vi "Think 3.vi"(2 "World (mapped) in":i8[][](array[numeric]), 3 "E":i8, 4 "Sense Heading":i8, 5 "Sensor View":i8[][](array[numeric]), 6 "Y":i8, 7 "X":i8) -> (0 "World (mapped) out":i8[][](array[numeric]), 1 "V Heading":i8)   [LabVIEW 2014]
doc: "This VI takes in the current location of the robot (X,Y), the 3x3 sensor reading of the surrounding area, and the direction of the highest-valued neighboring food source."
uses:
  <vilib>/imath/engines/lvmath2/RunTimeEngine/BuiltInFunctions/findnz/NIMS_[3o]_findnz(GM).vi
  <instcachedir>/0/NIMS_[3o]_findnz(GM)_AD3DA0EED2E643EC9DE9AF9EC032A43D.lvgen/NIMS_[3o]_findnz(GM)_AD3DA0EED2E643EC9DE9AF9EC032A43D_003.vi
  <vilib>/imath/engines/lvmath2/RunTimeEngine/BuiltInFunctions/length/NIMS_length(GM).vi
  <instcachedir>/0/NIMS_length(GM)_47CEC356FCE0482D9BA47DC61C99F2C7.lvgen/NIMS_length(GM)_47CEC356FCE0482D9BA47DC61C99F2C7_001.vi
  <vilib>/imath/engines/lvmath2/RunTimeEngine/RangeToken/NIMS_Range_R2 - Integer.vi
  <instcachedir>/0/NIMS_Range_R2 - Integer_2D1304BAF97744E0A293025746CBADFC.lvgen/NIMS_Range_R2 - Integer_2D1304BAF97744E0A293025746CBADFC_000.vi
  <vilib>/imath/engines/lvmath2/RunTimeEngine/CommandStatement/MC_CommandStatement_break.vi
  <vilib>/imath/engines/lvmath2/RunTimeEngine/VariableToken/NIMS_VariableToken_CondDefinedDefinedByReplace.vi
  <instcachedir>/0/NIMS_VariableToken_CondDefinedDefinedByReplace_D162CFFC24174562A9FEA619A91E1A56.lvgen/NIMS_VariableToken_CondDefinedDefinedByReplace_D162CFFC24174562A9FEA619A91E1A56_002.vi
  <vilib>/imath/engines/lvmath2/RunTimeEngine/IndexRead/NIMS M(S).vi
  <instcachedir>/0/NIMS M(S)_B826C018497E4940AE96BD27B540B6FB.lvgen/NIMS M(S)_B826C018497E4940AE96BD27B540B6FB_005.vi
  <vilib>/imath/engines/lvmath2/RunTimeEngine/IndexReplace/NIMS V(S)=S.vi
  <instcachedir>/0/NIMS V(S)=S_2D52C4EC15D8415E870AEE69FB516CCA.lvgen/NIMS V(S)=S_2D52C4EC15D8415E870AEE69FB516CCA_003.vi
  <vilib>/imath/engines/lvmath2/RunTimeEngine/ErrorHandling/NIMS_Create Error From Enums.vi
  <vilib>/imath/engines/lvmath2/RunTimeEngine/IndexRead/NIMS V(S).vi
  <instcachedir>/0/NIMS V(S)_0488751826AF41519A22953C041130DC.lvgen/NIMS V(S)_0488751826AF41519A22953C041130DC_002.vi
  <vilib>/imath/engines/lvmath2/RunTimeEngine/BuiltInFunctions/abs/NIMS_abs(signed).vi
  <instcachedir>/0/NIMS_abs(signed)_C4FCB8E6058B49B797C7C8D53CA5F6EC.lvgen/NIMS_abs(signed)_C4FCB8E6058B49B797C7C8D53CA5F6EC_007.vi
  <vilib>/imath/engines/lvmath2/RunTimeEngine/VariableToken/NIMS_VariableToken_CondDefined.vi
  <instcachedir>/0/NIMS_VariableToken_CondDefined_EE8DD211A89249938CE6537267F5C9B3.lvgen/NIMS_VariableToken_CondDefined_EE8DD211A89249938CE6537267F5C9B3_006.vi
  <vilib>/imath/engines/lvmath2/RunTimeEngine/BuiltInFunctions/min/1 input/NIMS_min(RV).vi
  <instcachedir>/0/NIMS_min(RV)_EE2DD3E2888846108C5160A664B67832.lvgen/NIMS_min(RV)_EE2DD3E2888846108C5160A664B67832_002.vi
  <vilib>/imath/engines/lvmath2/RunTimeEngine/BuiltInFunctions/findnz/NIMS_[1o]_findnz(GRowV).vi
  <instcachedir>/0/NIMS_[1o]_findnz(GRowV)_09DEEFCD766A4095B33095726AFD3FF8.lvgen/NIMS_[1o]_findnz(GRowV)_09DEEFCD766A4095B33095726AFD3FF8_000.vi
  <vilib>/imath/engines/lvmath2/RunTimeEngine/BuiltInFunctions/length/NIMS_length(GV).vi
  <instcachedir>/0/NIMS_length(GV)_08A3D13377FD4E4B96F5795FBF3698FA.lvgen/NIMS_length(GV)_08A3D13377FD4E4B96F5795FBF3698FA_002.vi
  <vilib>/imathl/engines/lvmath/Functions/Error Handling/Create Error.vi
  <vilib>/imath/engines/lvmath2/RunTimeEngine/IndexRead/NIMS M(V).vi
  <instcachedir>/0/NIMS M(V)_948FAC22C1C943948B75DA6190348614.lvgen/NIMS M(V)_948FAC22C1C943948B75DA6190348614_000.vi
  <vilib>/imath/engines/lvmath2/RunTimeEngine/NodeEndStatement/NIMS_NodeEndStatement_Output.vi
  <instcachedir>/0/NIMS_NodeEndStatement_Output_53EC0D466D134D7ABD903AC30B43404B.lvgen/NIMS_NodeEndStatement_Output_53EC0D466D134D7ABD903AC30B43404B_013.vi
  <vilib>/imath/engines/lvmath2/RunTimeEngine/ErrorHandling/NIMS_Finalize Error.vi
  <vilib>/imath/engines/lvmath2/RunTimeEngine/Managers/WorkSpace/UID Generator.vi
  <vilib>/imath/engines/lvmath2/RunTimeSupport/NIMS_Get Scalar_w Error.vi
  <instcachedir>/0/NIMS_Get Scalar_w Error_210488738D9D47B99AC00AB5D3B10099.lvgen/NIMS_Get Scalar_w Error_210488738D9D47B99AC00AB5D3B10099_007.vi
  <vilib>/imath/engines/lvmath2/RunTimeEngine/RunTimeType/NIMS_RunTimeType_From StrictType (excl LVString).vi
  <instcachedir>/0/NIMS_RunTimeType_From StrictType (excl LVString)_15A5391EEA9C4AACB9955AC755B83D29.lvgen/NIMS_RunTimeType_From StrictType (excl LVString)_15A5391EEA9C4AACB9955AC755B83D29_000.vi
  <vilib>/imath/engines/lvmath2/RunTimeEngine/LocalVariableDefStatement/MC_LocalVariableDefStatement_Display.vi
  <instcachedir>/0/NIMS_VariableToken_CondDefined_EE8DD211A89249938CE6537267F5C9B3.lvgen/NIMS_VariableToken_CondDefined_EE8DD211A89249938CE6537267F5C9B3_003.vi
  <vilib>/imath/engines/lvmath/Functions/Error Handling/MergeErrorsWrapper.vi
  <vilib>/imath/engines/lvmath2/RunTimeEngine/Managers/SymbolTable/Clear UID.vi
  <instcachedir>/0/NIMS_NodeEndStatement_Output_53EC0D466D134D7ABD903AC30B43404B.lvgen/NIMS_NodeEndStatement_Output_53EC0D466D134D7ABD903AC30B43404B_012.vi
  <instcachedir>/0/NIMS_NodeEndStatement_Output_53EC0D466D134D7ABD903AC30B43404B.lvgen/NIMS_NodeEndStatement_Output_53EC0D466D134D7ABD903AC30B43404B_011.vi
  <vilib>/imath/engines/lvmath2/RunTimeEngine/Managers/SymbolTable/NIMS_WorkSpace.lvlib
panel:
  out "Array":i8[](array[numeric])
  out "Numeric":dbl
  out "yrobot (unexplored)":i8
  out "xrobot (unexplored)":i8
  out "yrobot":i8
  out "xrobot":i8
  out "ytarget":i8
  out "xtarget":i8
  out "Mathscript Error (known target)":bool
  out "Array Index 1":i8
  out "Array Index 0":i8
  out "Array Size":i32
  # "Vcode\n  6 7 8\n  5 0 1\n  4 3 2"
  # "y"
  # "x"
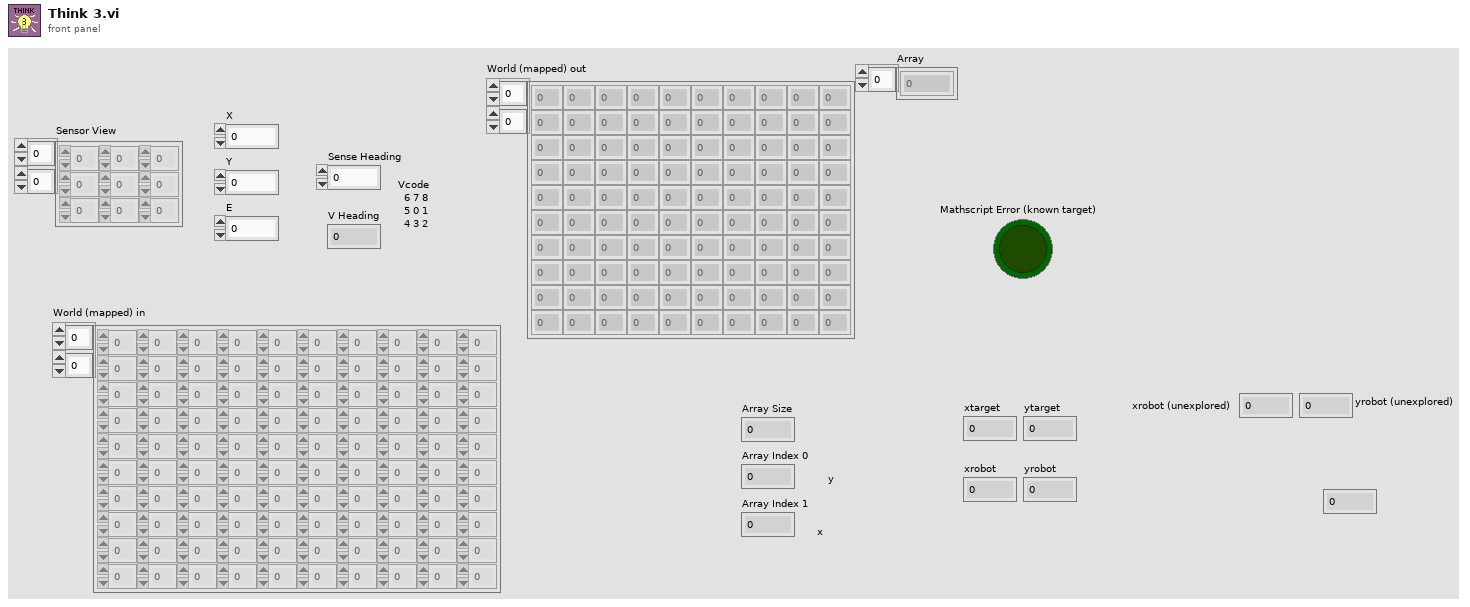
[diagram p1: front panel]
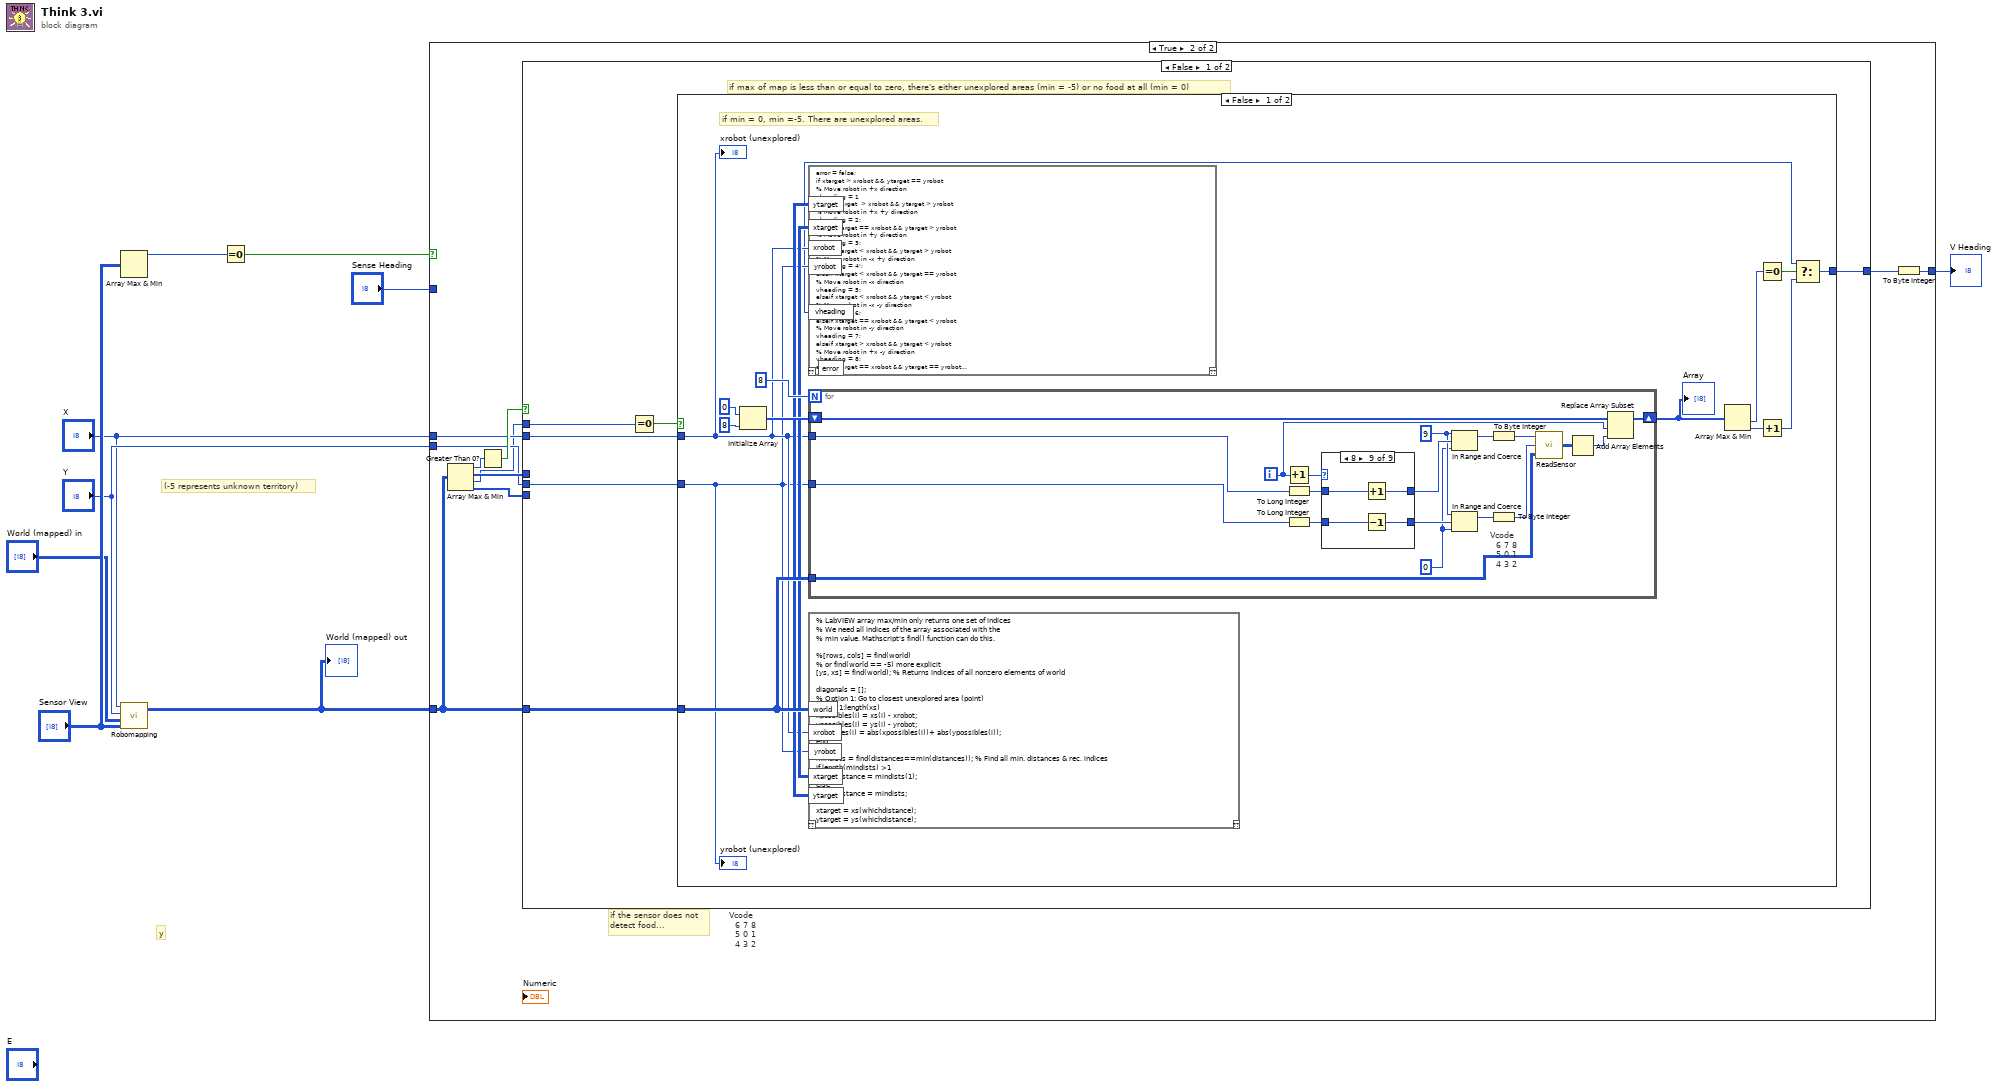
[diagram p0: block diagram]
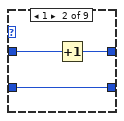
[diagram p4: hidden frame]
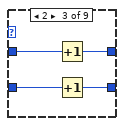
[diagram p5: hidden frame]
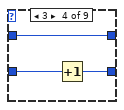
[diagram p6: hidden frame]
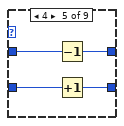
[diagram p7: hidden frame]
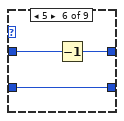
[diagram p8: hidden frame]
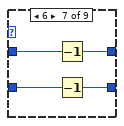
[diagram p9: hidden frame]
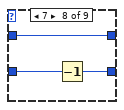
[diagram p10: hidden frame]
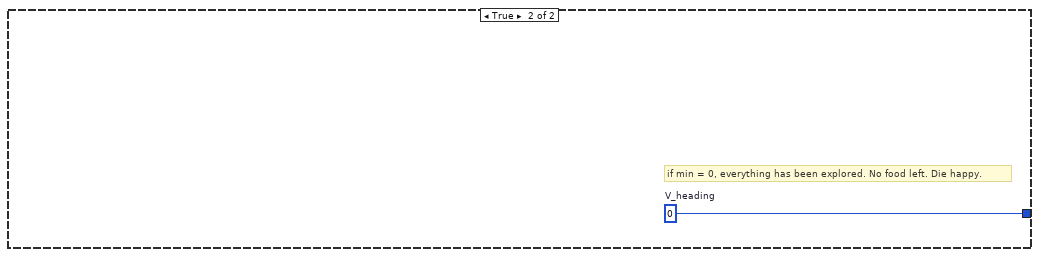
[diagram p11: hidden frame]
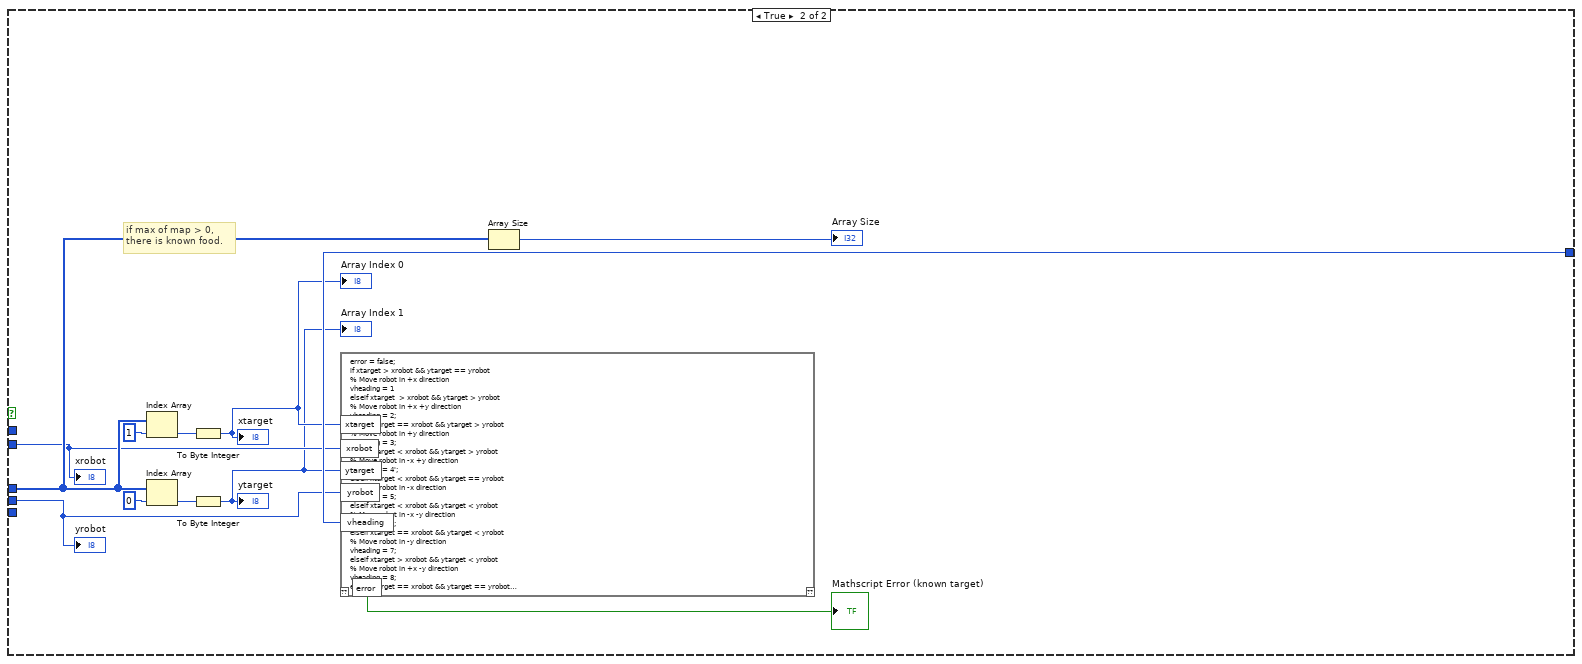
[diagram p12: hidden frame]
diagram:
  # "y"
  # "(-5 represents unknown territory)"
  n1 = Array Max & Min(array="Sensor View") -> (max value=w9:i8)  [unwired: 3 out]
  n2 = call "Robomapping.vi"("Sensor View"="Sensor View", "World (mapped) in"="World (mapped) in", "Y"="Y", "X"="X") -> ("World (mapped) out"=w1:i8[][])  [unwired: 1 out]
  "World (mapped) out" <- w1
  n3 = Equal To 0?(x=w9) -> (x = 0?=w8:bool)
  n4 = case shown="True" w8 {
    tunnel: "X" -> [_ w17]
    tunnel: "Y" -> [_ w16]
    tunnel: [w10 w11] -> w6
    tunnel: w1 -> [_ w12]
    tunnel: "Sense Heading" -> [w10 _]
    frame False {
      # "If the sensor detects food, use the sense heading"
    }
    frame True {
      # "if the sensor does not\ndetect food..."
      # "Vcode\n  6 7 8\n  5 0 1\n  4 3 2"
      n5 = Array Max & Min(array=w12) -> (max value=w20:i8, max index (indices)=w18:i32[], min value=w15:i8, min index (indices)=w14:i32[])
      n6 = Greater Than 0?(x=w20) -> (x > 0?=w19:bool)
      n7 = case shown="False" w19 {
        tunnel: w18 -> [_ w975]
        tunnel: w17 -> [w21 w967]
        tunnel: w16 -> [w22 w969]
        tunnel: [w24 w971] -> w13
        tunnel: w15 -> [w25 _]
        tunnel: w14 -> [_ _]
        tunnel: w12 -> [w23 _]
        frame False {
          # "if max of map is less than or equal to zero, there's either unexplored areas (min = -5) or no food at all (min = 0)"
          n8 = Equal To 0?(x=w25) -> (x = 0?=w26:bool)
          n9 = case shown="False" w26 {
            tunnel: [w33 w965] -> w24
            tunnel: w23 -> [w32 _]
            tunnel: w21 -> [w29 _]
            tunnel: w22 -> [w28 _]
            frame False {
              # "if min = 0, min =-5. There are unexplored areas."
              n10 = Initialize Array(i8 0 ("element"), 8 ("dimension size")) -> (w39:i8[])
              n11 = for {
                N: 8 -> [_]
                tunnel: w29 -> [w930]
                tunnel: w28 -> [w929]
                tunnel: w32 -> [w922]
                shift-right: [w918] -> w40
                shift-left: w39 -> [w919]
                i -> [w916]
                w931 = 0
                w932 = 9
                # "Vcode\n  6 7 8\n  5 0 1\n  4 3 2"
                n12 = Increment(x=w916) -> (x+1=w920:i32)
                n13 = To Long Integer(number=w930) -> (32bit integer=w928:i32)
                n14 = To Long Integer(number=w929) -> (32bit integer=w927:i32)
                n15 = case shown="8" w920 {
                  tunnel: w928 -> [w935 w939 w943 w944 w947 w953 w957 w958 w964]
                  tunnel: w927 -> [w936 w937 w941 w946 w950 w951 w955 w960 w962]
                  tunnel: [w935 w938 w942 w944 w948 w952 w956 w958 w963] -> w934
                  tunnel: [w936 w937 w940 w945 w949 w951 w954 w959 w961] -> w933
                  frame 0, Default {
                  }
                  frame 1 {
                    n16 = Increment(x=w939) -> (x+1=w938:i32)
                  }
                  frame 2 {
                    n17 = Increment(x=w943) -> (x+1=w942:i32)
                    n18 = Increment(x=w941) -> (x+1=w940:i32)
                  }
                  frame 3 {
                    n19 = Increment(x=w946) -> (x+1=w945:i32)
                  }
                  frame 4 {
                    n20 = Decrement(x=w947) -> (x-1=w948:i32)
                    n21 = Increment(x=w950) -> (x+1=w949:i32)
                  }
                  frame 5 {
                    n22 = Decrement(x=w953) -> (x-1=w952:i32)
                  }
                  frame 6 {
                    n23 = Decrement(x=w957) -> (x-1=w956:i32)
                    n24 = Decrement(x=w955) -> (x-1=w954:i32)
                  }
                  frame 7 {
                    n25 = Decrement(x=w960) -> (x-1=w959:i32)
                  }
                  frame 8 {
                    n26 = Increment(x=w964) -> (x+1=w963:i32)
                    n27 = Decrement(x=w962) -> (x-1=w961:i32)
                  }
                }
                n28 = In Range and Coerce(upper limit=w932, x=w934, lower limit=w931) -> (coerced(x)=w926:i32)  [unwired: 1 out]
                n29 = In Range and Coerce(upper limit=w932, x=w933, lower limit=w931) -> (coerced(x)=w925:i32)  [unwired: 1 out]
                n30 = To Byte Integer(number=w926) -> (8bit integer=w923:i8)
                n31 = To Byte Integer(number=w925) -> (8bit integer=w924:i8)
                n32 = call "ReadSensor.vi"("World"=w922, "Y"=w924, "X"=w923) -> ("Sensor Array"=w921:i8[][])
                n33 = Add Array Elements(numeric array=w921) -> (sum=w917:i8)
                n34 = Replace Array Subset(array=w919, new element=w917, index=w916) -> (w918:i8[])
              }
              "Array" <- w40
              n35 = mathscript code="% LabVIEW array max/min only returns one set of indices\n% We need all indices of the array associated with the\n% min value. Mathscript's find() function can do this.\n\n%[rows, cols] = find(world)\n% or find(world == -5) more explicit\n[ys, xs] = find(world); % Returns indices of all nonzero elements of world\n \ndiagonals = [];\n% Option 1: Go to closest unexplored area (point)\nfor i = 1:length(xs)\nxpossibles(i) = xs(i) - xrobot;\nypossibles(i) = ys(i) - yrobot;\ndistances(i) = abs(xpossibles(i))+ abs(ypossibles(i));\nend\n\nmindists = find(distances==min(distances)); % Find all min. distances & rec. indices\nif length(mindists) >1\nwhichdistance = mindists(1);\nelse\nwhichdistance = mindists;\nend\nxtarget = xs(whichdistance);\nytarget = ys(whichdistance);\n\n\n% Option 2: Go towards average of unexplored points\n% BAD\n%xavg = mean(xs);\n%yavg = mean(ys);\n%xtarget = xavg;\n%ytarget = yavg; \n\n% Option 3: Go towards mode of unexplored points\n\n% mode fxn doesn't work..."("world"=w32, "xrobot"=w29, "yrobot"=w28) -> ("ytarget"=w30:i32[][], "xtarget"=w31:i32[][])  [unwired: 1 in, 1 out]
              n36 = mathscript code="error = false;\nif xtarget > xrobot && ytarget == yrobot\n% Move robot in +x direction\nvheading = 1\nelseif xtarget  > xrobot && ytarget > yrobot\n% Move robot in +x +y direction\nvheading = 2;\nelseif xtarget == xrobot && ytarget > yrobot\n% Move robot in +y direction\nvheading = 3;\nelseif xtarget < xrobot && ytarget > yrobot\n% Move robot in -x +y direction\nvheading = 4';\nelseif xtarget < xrobot && ytarget == yrobot\n% Move robot in -x direction\nvheading = 5;\nelseif xtarget < xrobot && ytarget < yrobot\n% Move robot in -x -y direction\nvheading = 6;\nelseif xtarget == xrobot && ytarget < yrobot\n% Move robot in -y direction\nvheading = 7;\nelseif xtarget > xrobot && ytarget < yrobot\n% Move robot in +x -y direction\nvheading = 8;\nelseif xtarget == xrobot && ytarget == yrobot\n% This shouldn't happen. Included for completeness & debugging\nvheading = 0;\nerror = true;\nend"("xtarget"=w31, "yrobot"=w28, "xrobot"=w29, "ytarget"=w30) -> ("vheading"=w27:i32)  [unwired: 1 in, 2 out]
              n37 = Array Max & Min(array=w40) -> (min value=w35:i8, min index (indices)=w41:i32)  [unwired: 2 out]
              n38 = Equal To 0?(x=w35) -> (x = 0?=w36:bool)
              n39 = Increment(x=w41) -> (x+1=w34:i32)
              n40 = Select(t=w27, s=w36, f=w34) -> (s? t:f=w33:i32)
              "xrobot (unexplored)" <- w29
              "yrobot (unexplored)" <- w28
            }
            frame True {
              w965 = 0  # V_heading
              # "if min = 0, everything has been explored. No food left. Die happy."
            }
          }
        }
        frame True {
          # "if max of map > 0,\nthere is known food."
          n41 = Index Array ("x index")(array=w975, index=1) -> (element=w972:i32)
          n42 = Index Array ("y index")(array=w975, index=0) -> (element=w973:i32)
          n43 = To Byte Integer(number=w972) -> (8bit integer=w968:i8)
          "Array Index 0" <- w968
          "xtarget" <- w968
          n44 = To Byte Integer(number=w973) -> (8bit integer=w966:i8)
          "Array Index 1" <- w966
          "ytarget" <- w966
          n45 = mathscript code="error = false;\nif xtarget > xrobot && ytarget == yrobot\n% Move robot in +x direction\nvheading = 1\nelseif xtarget  > xrobot && ytarget > yrobot\n% Move robot in +x +y direction\nvheading = 2;\nelseif xtarget == xrobot && ytarget > yrobot\n% Move robot in +y direction\nvheading = 3;\nelseif xtarget < xrobot && ytarget > yrobot\n% Move robot in -x +y direction\nvheading = 4';\nelseif xtarget < xrobot && ytarget == yrobot\n% Move robot in -x direction\nvheading = 5;\nelseif xtarget < xrobot && ytarget < yrobot\n% Move robot in -x -y direction\nvheading = 6;\nelseif xtarget == xrobot && ytarget < yrobot\n% Move robot in -y direction\nvheading = 7;\nelseif xtarget > xrobot && ytarget < yrobot\n% Move robot in +x -y direction\nvheading = 8;\nelseif xtarget == xrobot && ytarget == yrobot\n% This shouldn't happen. Included for completeness & debugging\nvheading = 0;\nerror = true;\nend"("xtarget"=w968, "yrobot"=w969, "xrobot"=w967, "ytarget"=w966) -> ("vheading"=w971:i32, "error"=→"Mathscript Error (known target)":bool)  [unwired: 1 in, 1 out]
          n46 = Array Size(array=w975) -> (size(s)=→"Array Size":i32)
          "xrobot" <- w967
          "yrobot" <- w969
        }
      }
      n47 = To Byte Integer(number=w13) -> (8bit integer=w11:i8)
    }
  }
  "V Heading" <- w6
